vi "GetHigherBound.vi"(8 "error in":errorcluster, 11 "DateTimeMeasureLimit in":refnum<class "DateTimeMeasureLimit.lvclass">) -> (0 "error out":errorcluster, 2 "HigherBound":timestamp, 3 "DateTimeMeasureLimit out":refnum<class "DateTimeMeasureLimit.lvclass">)   [LabVIEW 2021, in "ProligentXMLGenerator.lvlib" / "DateTimeMeasureLimit.lvclass"]
doc: "Real Measure Limit Higher Bound"
uses:
  DateTimeMeasureLimit.lvclass
  DateTimeMeasureLimit.lvclass/DateTimeMeasureLimit.ctl
  Base/DateTime/DateTime.lvclass
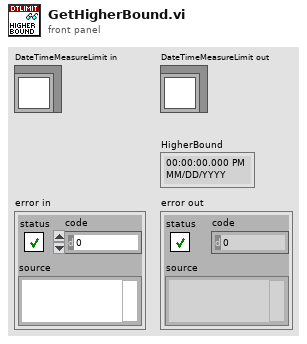
[diagram p1: front panel]
types:
  T1 = typedef "ProligentXMLGenerator.lvlib/DateTimeMeasureLimit.lvclass/Data.ctl" = cluster{"LowerBound":refnum<class "DateTime.lvclass">, "HigherBound":refnum<class "DateTime.lvclass">}
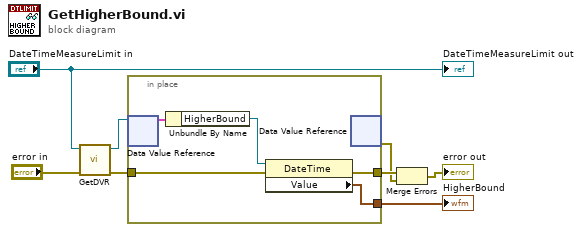
[diagram p0: block diagram]
diagram:
  n1 = call "GetDVR.vi"("error in"="error in", "DateTimeMeasureLimit"="DateTimeMeasureLimit in") -> ("error out"=w6:errorcluster, "DVRReference"=w5:refnum<data-value>)  [unwired: 8 in]
  n2 = in-place "In Place Element Structure" {
    in-place-border: [w9] -> w1
    in-place-border: w6 -> [w11]
    in-place-border: [w10] -> w4
    n3 = in-place-dvr #1(w5) -> (w13:T1)  [unwired: 1 out]
    n4 = Unbundle By Name(w13) -> ("HigherBound"=w12:refnum<class "DateTime.lvclass">)
    n5 = property class="DateTime"(reference=w12, error in=w11) -> (error out=w10:errorcluster, "Value"=w9:timestamp)  [unwired: 1 out]
    n6 = in-place-dvr #1() -> (w2:errorcluster)  [unwired: 1 in, 1 out]
  }
  "HigherBound" <- w1
  n7 = Merge Errors(w4, w2) -> (→"error out":errorcluster)
  "DateTimeMeasureLimit out" <- "DateTimeMeasureLimit in"
